vi "LaunchDependency.vi"(6 "Shared Resource":bool, 8 "error in (no error)":errorcluster, 9 "Dependency Name":string, 10 "Dependency Type":refnum<class "SMO.lvclass">, 11 "SMO in":refnum<class "SMO.lvclass">) -> (0 "error out":errorcluster, 1 "Unique Name":string, 2 "Dependency Reference":refnum<class "SMO.lvclass">, 3 "SMO out":refnum<class "SMO.lvclass">)   [LabVIEW 2021, in "smo.lvlib" / "SMO.lvclass"]
doc: "This method allows the SMO to launch a dependency and take ownership of its lifetime through composition (if not already owned) or add it to its dependencies' list through aggregation (if owned by another subsystem).\n\nA SMO that is owned by another SMO means that its lifetime is managed by the dependee. When the top-level SMO stops or gets destroyed, the owned dependencies will also be stopped or destroyed in the process.\n\nA SMO that aggregates another SMO, but does not own it, will be unable to change the state of the subsystem because its lifetime is managed by its owner.\n\n\"Dependency Name\" is the equivalent of \"Subsystem Name\" for the Create method, but for the Dependency.\n\n\"Dependency Type\" can be an uninitialized SMO object or an already created object.\nIf the input is not yet a constructed SMO, the object type is used, by value, to Create a new SMO instance of this class. On the contrary, if the Dependency Type is an already constructed or started SMO, the creation and/or start process is skipped. The caller SMO will always request to take ownership of the SMO dependency. If it is not already owned by another subsystem, the caller will succeed in taking ownership, and from this time forward, will manage the lifetime of the dependency.\n\n\"Dependency Reference\" is the created SMO instance and can be interacted with through the public API, like any normal SMO on a block diagram."
uses:
  SMO.lvclass
  SMO.lvclass/SMO.ctl
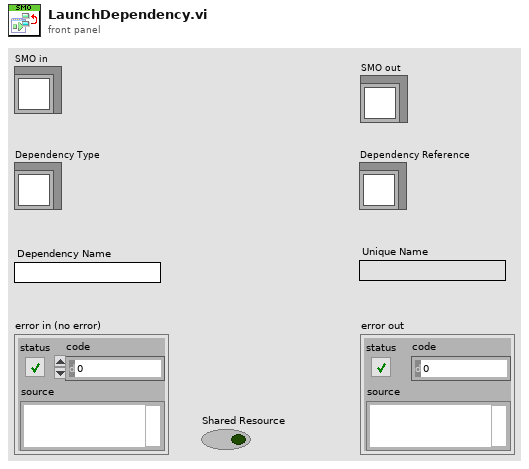
[diagram p1: front panel]
types:
  T1 = typedef "smo.lvlib/SMO.lvclass/SMOState --Enum.ctl" = enum16{"unknown", "Created", "Started", "Stopped"}
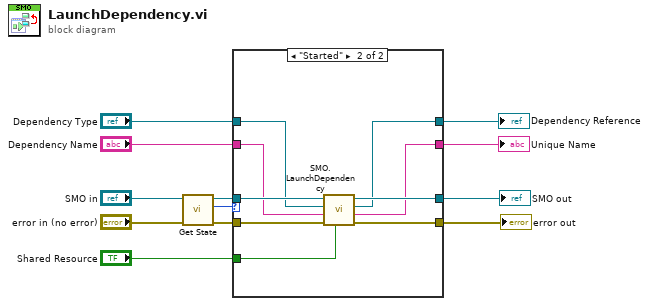
[diagram p0: block diagram]
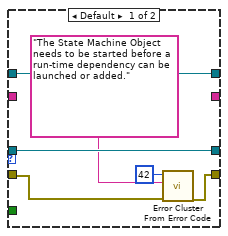
[diagram p2: hidden frame]
diagram:
  n1 = call "Get State.vi"("error in (no error)"="error in (no error)", "SMO"="SMO in") -> ("error out"=w9:errorcluster, "SMO State"=w6:T1, "SMO out"=w11:refnum<class "SMO.lvclass">)  [unwired: 7 in]
  n2 = case shown="\"Started\"" w6 {
    tunnel: w11 -> [w18 w27]
    tunnel: [w18 w26] -> w10
    tunnel: w9 -> [w16 w25]
    tunnel: [w17 w24] -> w7
    tunnel: "Dependency Type" -> [w13 w23]
    tunnel: "Dependency Name" -> [_ w22]
    tunnel: [_ w21] -> w3
    tunnel: "Shared Resource" -> [_ w20]
    tunnel: [w13 w19] -> w1
    frame Default {
      n3 = call <vilib>:"Error Cluster From Error Code.vi"("error in (no error)"=w16, "error message (\"\")"="The State Machine Object needs to be started before a run-time dependency can be launched or added." ("error message (\"\")"), "error code (0)"=42) -> ("error out"=w17:errorcluster)  [unwired: 6 in]
    }
    frame "Started" {
      n4 = call "SMO.LaunchDependency.vi"("Shared Resource"=w20, "error in (no error)"=w25, "Dependency Name"=w22, "Dependency Type"=w23, "SMO in"=w27) -> ("error out"=w24:errorcluster, "Unique Name"=w21:string, "Dependency Reference"=w19:refnum<class "SMO.lvclass">, "SMO out"=w26:refnum<class "SMO.lvclass">)  [unwired: 3 in]
    }
  }
  "error out" <- w7
  "SMO out" <- w10
  "Unique Name" <- w3
  "Dependency Reference" <- w1
